vi "Teleop.vi"(10 "Match Info":T1={"Autonomous Elapsed Seconds"=0.0, "TeleOp Elapsed Seconds"=0.0, "Disabled Elapsed Seconds"=0.0, "Visited Autonomous"=FALSE, "Visited TeleOp"=FALSE, "Visited Disabled"=FALSE, "Autonomous Settings"={"Autonomous Style"=enum."Independent", "VI Refnum"=refnum}}, 11 "Call Context":T2) -> ()   [LabVIEW 2013]
doc: "This VI is called for each TeleOp packet received from the DS where the robot is not disabled. It is often used to read from the joysticks and update I/O or to update setpoints for timed control loops. It should complete and return within 20 milliseconds or it may miss DS packets."
uses:
  <vilib>/Rock Robotics/WPI/DriverStation/WPI_DriverStationDerivedRobotMode.ctl
  <vilib>/Rock Robotics/WPI/DriverStation/WPI_DriverStationMatch Info.ctl
  Robot Global Data.vi
  <vilib>/Rock Robotics/WPI/Joystick/WPI_JoystickGetSetRefNum.vi
  <vilib>/Rock Robotics/WPI/RobotDrive/WPI_RobotDriveGetSetRefNum.vi
panel:
  in  "last switch 2":bool
  in  "toggle on/off internal 2":bool=TRUE
  out "toggle on/off 2":bool=TRUE
  out "axis 1 (x) 2":dbl
  out "axis 2 (y) 2":dbl
  out "toggle on/off":bool=TRUE
  in  "toggle on/off internal":bool=TRUE
  in  "last switch":bool
  out "axis 1 (x)":dbl
  out "axis 2 (y)":dbl
  out "Numeric 1":dbl(slide) scale=0.0..100.0
  out "Boolean 2":bool
  out "Boolean 1":bool
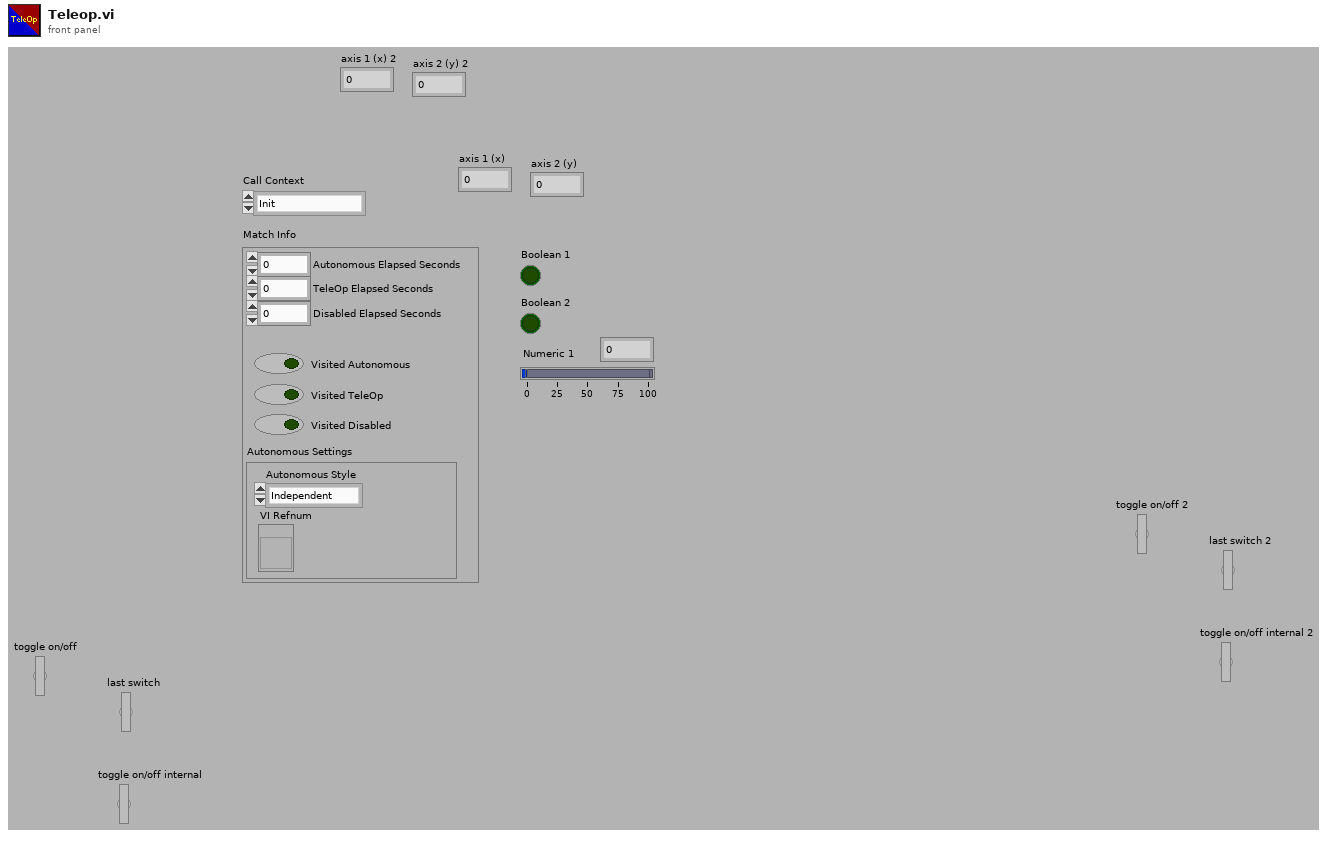
[diagram p1: front panel]
types:
  T1 = typedef "WPI_DriverStationMatch Info.ctl" = cluster{"Autonomous Elapsed Seconds":dbl, "TeleOp Elapsed Seconds":dbl, "Disabled Elapsed Seconds":dbl, "Visited Autonomous":bool, "Visited TeleOp":bool, "Visited Disabled":bool, "Autonomous Settings":cluster{"Autonomous Style":enum16{"Iterative", "Independent"}, "VI Refnum":refnum<vi>}}
  T2 = typedef "WPI_DriverStationDerivedRobotMode.ctl" = enum16{"Init", "Execute", "Stop"}
  T3 = typedef "WPI_JoystickDevRef.ctl" = cluster{"Device":T4}
  T4 = typedef "WPI_JoystickDeviceEnum.ctl" = enum16{"USB 1", "USB 2", "USB 3", "USB 4", "Kinect 1", "Kinect 2"}
  T5 = typedef "WPI_JoystickButtonState.ctl" = cluster{"Button 1":bool, "Button 2":bool, "Button 3":bool, "Button 4":bool, "Button 5":bool, "Button 6":bool, "Button 7":bool, "Button 8":bool, "Button 9":bool, "Button 10":bool, "Button 11":bool, "Button 12":bool}
  T6 = typedef "WPI_RobotDriveDevRef.ctl" = cluster{"DevStatus":errorcluster, "Motors[]":T7[], "Square Inputs":bool, "Max Output":dbl, "Isochronous":bool}
  T7 = typedef "WPI_MotorControlDeviceRef.ctl" = cluster{"DeviceStatus":errorcluster, "Type":enum16{"PWM", "CAN"}, "PWM":cluster{"Digital Module":T8, "PWM Channel":T9, "DeadBand":T10}, "CAN":cluster{"Device Number":u8, "Control Mode":T11, "Semaphore":T12, "Max Vout":dbl}, "Invert":bool, "TransformRef":T13, "InvTransformRef":T13}
  T8 = typedef "FPGA_TypedefDigitalModule.ctl" = enum16{"Digital Module 1", "Digital Module 2"}
  T9 = typedef "FPGA_DIOPWMChannel.ctl" = enum8{"PWM 1", "PWM 2", "PWM 3", "PWM 4", "PWM 5", "PWM 6", "PWM 7", "PWM 8", "PWM 9", "PWM 10", "Invalid"}
  T10 = typedef "WPI_PWMDeadband.ctl" = cluster{"Name":string, "maxPositivePwm":i32, "minPositivePwm":i32, "centerPwm":i32, "maxNegativePwm":i32, "minNegativePwm":i32, "angularRange":u16}
  T11 = typedef "WPI_CANJaguar_ControlMode.ctl" = enum8{"Percent VBus", "Current", "Speed", "Position", "Voltage"}
  T12 = typedef "Semaphore RefNum" = refnum<k1>
  T13 = typedef "WPI_PWMTransform_ConPane.ctl" = refnum<vi>
  T14 = cluster{"axis 1 (x)":dbl, "axis 2 (y)":dbl, "axis 3 (throttle)":dbl, "axis 4":dbl, "axis 5":dbl, "axis 6":dbl}
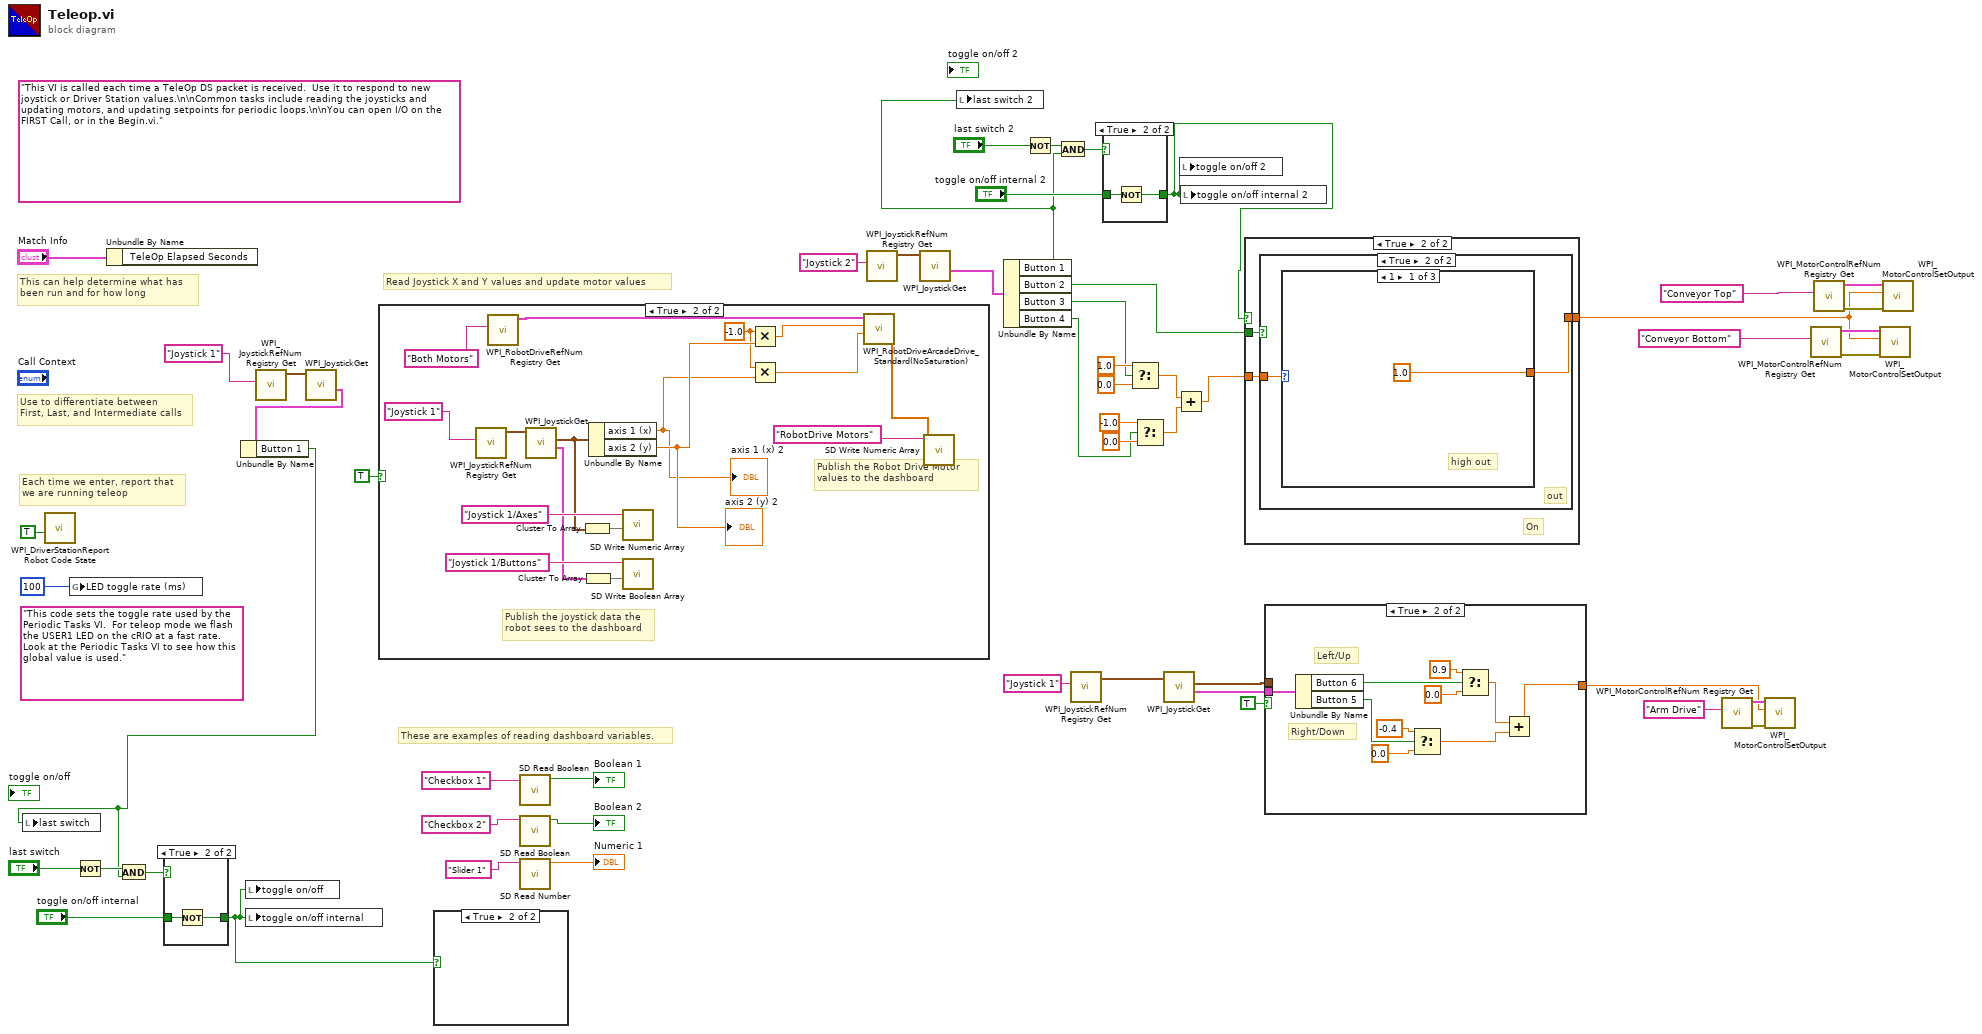
[diagram p0: block diagram]
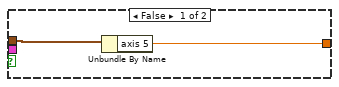
[diagram p3: hidden frame]
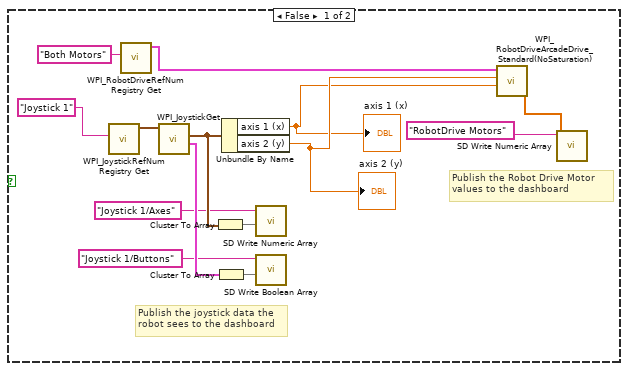
[diagram p6: hidden frame]
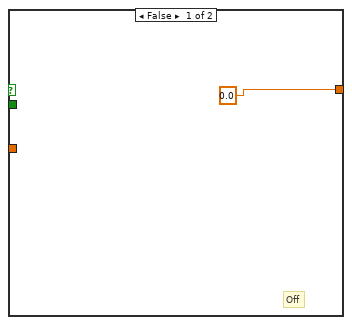
[diagram p7: hidden frame]
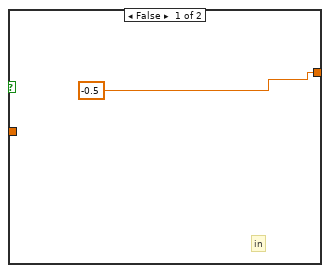
[diagram p8: hidden frame]
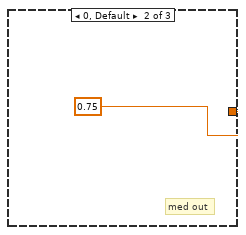
[diagram p9: hidden frame]
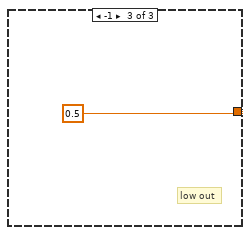
[diagram p10: hidden frame]
diagram:
  (unwired) "This code sets the toggle rate used by the Periodic Tasks VI.  For teleop mode we flash the USER1 LED on the cRIO at a fast rate.  Look at the Periodic Tasks VI to see how this global value is used."
  (unwired) "This VI is called each time a TeleOp DS packet is received.  Use it to respond to new joystick or Driver Station values.\n\nCommon tasks include reading the joysticks and updating motors, and updating setpoints for periodic loops.\n\nYou can open I/O on the FIRST Call, or in the Begin.vi."
  # "These are examples of reading dashboard variables."
  # "Each time we enter, report that\nwe are running teleop"
  # "Use to differentiate between\nFirst, Last, and Intermediate calls"
  # "This can help determine what has\nbeen run and for how long"
  # "Read Joystick X and Y values and update motor values"
  n1 = call <vilib>:"WPI_DriverStationReport Robot Code State.vi"("TeleOp"=TRUE ("Autonomous")) -> ()  [unwired: 10 in, 1 out]
  n2 = global write "Robot Global Data.vi" "LED toggle rate (ms)"(u32 100 ("LED ms toggle rate")) -> ()
  n3 = Not(x="last switch") -> (.not. x?=w25:bool)
  n4 = Unbundle By Name("Match Info") -> ()  [unwired: 1 out]
  n5 = call <vilib>:"WPI_JoystickRefNum Registry Get.vi"("refnum name"="Joystick 1") -> ("JoystickDevRef"=w29:T3)  [unwired: 1 in, 9 out]
  n6 = call <vilib>:"WPI_JoystickGet.vi"("JoystickDevRef"=w29) -> ("Buttons"=w27:T5)  [unwired: 1 in, 5 out]
  n7 = Unbundle By Name(w27) -> ("Button 1"=w22:bool)
  n8 = local write "last switch"(w22) -> ()
  n9 = And(x=w25, y=w22) -> (x .and. y?=w24:bool)
  n10 = case shown="True" w24 {
    tunnel: "toggle on/off internal" -> [w55 w57]
    tunnel: [w55 w56] -> w13
    frame False {
    }
    frame True {
      n11 = Not(x=w57) -> (.not. x?=w56:bool)
    }
  }
  n12 = local write "toggle on/off"(w13) -> ()
  n13 = local write "toggle on/off internal"(w13) -> ()
  n14 = case shown="True" TRUE {
    frame False {
      # "Publish the Robot Drive Motor\nvalues to the dashboard"
      # "Publish the joystick data the\nrobot sees to the dashboard"
      n15 = call <vilib>:"WPI_JoystickRefNum Registry Get.vi"("refnum name"="Joystick 1") -> ("JoystickDevRef"=w70:T3)  [unwired: 1 in, 9 out]
      n16 = call <vilib>:"WPI_RobotDriveRefNum Registry Get.vi"("refnum name"="Both Motors") -> ("RobotDriveDevRef"=w60:T6)  [unwired: 9 in, 1 out]
      n17 = call <vilib>:"WPI_JoystickGet.vi"("JoystickDevRef"=w70) -> ("Buttons"=w69:T5, "Axes"=w66:T14)  [unwired: 1 in, 4 out]
      n18 = Cluster To Array(cluster=w66) -> (array=w65:dbl[])
      n19 = Cluster To Array(cluster=w69) -> (array=w68:bool[])
      n20 = Unbundle By Name(w66) -> ("axis 1 (x)"=w58:dbl, "axis 2 (y)"=w59:dbl)
      "axis 2 (y)" <- w59
      "axis 1 (x)" <- w58
      n21 = call <vilib>:"SD Write Numeric Array.vi"("Numeric Array"=w65, "Name"="Joystick 1/Axes") -> ()  [unwired: 8 in, 2 out]
      n22 = call <vilib>:"SD Write Boolean Array.vi"("Boolean Array"=w68, "Name"="Joystick 1/Buttons") -> ()  [unwired: 8 in, 2 out]
      n23 = call <vilib>:"WPI_RobotDriveArcadeDrive_Standard(NoSaturation).vi"("Y axis value"=w58, "X axis value"=w59, "RobotDriveDevRef"=w60) -> ("Motor Values"=w62:dbl[])  [unwired: 1 in, 7 out]
      n24 = call <vilib>:"SD Write Numeric Array.vi"("Numeric Array"=w62, "Name"="RobotDrive Motors") -> ()  [unwired: 8 in, 2 out]
    }
    frame True {
      w73 = -1.0 ("x")
      # "Publish the Robot Drive Motor\nvalues to the dashboard"
      # "Publish the joystick data the\nrobot sees to the dashboard"
      n25 = call <vilib>:"WPI_JoystickRefNum Registry Get.vi"("refnum name"="Joystick 1") -> ("JoystickDevRef"=w78:T3)  [unwired: 1 in, 9 out]
      n26 = call <vilib>:"WPI_RobotDriveRefNum Registry Get.vi"("refnum name"="Both Motors") -> ("RobotDriveDevRef"=w88:T6)  [unwired: 9 in, 1 out]
      n27 = call <vilib>:"WPI_JoystickGet.vi"("JoystickDevRef"=w78) -> ("Buttons"=w79:T5, "Axes"=w82:T14)  [unwired: 1 in, 4 out]
      n28 = Cluster To Array(cluster=w82) -> (array=w83:dbl[])
      n29 = Cluster To Array(cluster=w79) -> (array=w80:bool[])
      n30 = Unbundle By Name(w82) -> ("axis 1 (x)"=w72:dbl, "axis 2 (y)"=w76:dbl)
      "axis 2 (y) 2" <- w76
      "axis 1 (x) 2" <- w72
      n31 = call <vilib>:"SD Write Numeric Array.vi"("Numeric Array"=w83, "Name"="Joystick 1/Axes") -> ()  [unwired: 8 in, 2 out]
      n32 = call <vilib>:"SD Write Boolean Array.vi"("Boolean Array"=w80, "Name"="Joystick 1/Buttons") -> ()  [unwired: 8 in, 2 out]
      n33 = Multiply(x=w73, y=w76) -> (x*y=w75:dbl)
      n34 = Multiply(x=w73, y=w72) -> (x*y=w74:dbl)
      n35 = call <vilib>:"WPI_RobotDriveArcadeDrive_Standard(NoSaturation).vi"("Y axis value"=w74, "X axis value"=w75, "RobotDriveDevRef"=w88) -> ("Motor Values"=w86:dbl[])  [unwired: 1 in, 7 out]
      n36 = call <vilib>:"SD Write Numeric Array.vi"("Numeric Array"=w86, "Name"="RobotDrive Motors") -> ()  [unwired: 8 in, 2 out]
    }
  }
  n37 = case shown="True" w13 {
    frame False {
    }
    frame True {
    }
  }
  n38 = call <vilib>:"SD Read Boolean.vi"("Name"="Checkbox 1" ("refnum name")) -> ("Boolean"=→"Boolean 1":bool)  [unwired: 8 in, 2 out]
  n39 = call <vilib>:"SD Read Boolean.vi"("Name"="Checkbox 2" ("refnum name")) -> ("Boolean"=→"Boolean 2":bool)  [unwired: 8 in, 2 out]
  n40 = call <vilib>:"SD Read Number.vi"("Name"="Slider 1" ("refnum name")) -> ("Numeric"=→"Numeric 1":dbl)  [unwired: 8 in, 2 out]
  n41 = call <vilib>:"WPI_JoystickRefNum Registry Get.vi"("refnum name"="Joystick 2") -> ("JoystickDevRef"=w39:T3)  [unwired: 9 in, 1 out]
  n42 = call <vilib>:"WPI_JoystickGet.vi"("JoystickDevRef"=w39) -> ("Buttons"=w37:T5)  [unwired: 4 in, 2 out]
  n43 = Unbundle By Name(w37) -> ("Button 1"=w4:bool, "Button 2"=w14:bool, "Button 3"=w1:bool, "Button 4"=w2:bool)
  n44 = local write "last switch 2"(w4) -> ()
  n45 = Not(x="last switch 2") -> (.not. x?=w6:bool)
  n46 = And(x=w6, y=w4) -> (x .and. y?=w7:bool)
  n47 = call <vilib>:"WPI_JoystickRefNum Registry Get.vi"("refnum name"="Joystick 1") -> ("JoystickDevRef"=w44:T3)  [unwired: 9 in, 1 out]
  n48 = case shown="True" w7 {
    tunnel: "toggle on/off internal 2" -> [w89 w91]
    tunnel: [w89 w90] -> w3
    frame False {
    }
    frame True {
      n49 = Not(x=w91) -> (.not. x?=w90:bool)
    }
  }
  n50 = Select(t=1.0, s=w1, f=0.0) -> (s? t:f=w16:dbl)
  n51 = Select(t=-1.0, s=w2, f=0.0) -> (s? t:f=w17:dbl)
  n52 = call <vilib>:"WPI_JoystickGet.vi"("JoystickDevRef"=w44) -> ("Buttons"=w43:T5, "Axes"=w10:T14)  [unwired: 4 in, 1 out]
  n53 = Add(x=w16, y=w17) -> (x+y=w15:dbl)
  n54 = local write "toggle on/off 2"(w3) -> ()
  n55 = local write "toggle on/off internal 2"(w3) -> ()
  n56 = case shown="True" w3 {
    tunnel: [0.0 ("f") w94] -> w30
    tunnel: w15 -> [_ w95]
    tunnel: w14 -> [_ w93]
    frame False {
      # "Off"
    }
    frame True {
      # "On"
      n57 = case shown="True" w93 {
        tunnel: w95 -> [_ w98]
        tunnel: [-0.5 ("t") w97] -> w94
        frame False {
          # "in"
        }
        frame True {
          # "out"
          n58 = case shown="1" w98 {
            tunnel: [1.0 ("t") 0.75 ("t") 0.5 ("f")] -> w97
            frame 1 {
              # "high out"
            }
            frame 0, Default {
              # "med out"
            }
            frame -1 {
              # "low out"
            }
          }
        }
      }
    }
  }
  n59 = case shown="True" TRUE {
    tunnel: w43 -> [_ w113]
    tunnel: w10 -> [w103 _]
    tunnel: [w102 w104] -> w9
    frame False {
      n60 = Unbundle By Name(w103) -> ("axis 5"=w102:dbl)
    }
    frame True {
      # "Right/Down"
      # "Left/Up"
      n61 = Unbundle By Name(w113) -> ("Button 6"=w112:bool, "Button 5"=w111:bool)
      n62 = Select(t=-0.4, s=w111, f=0.0) -> (s? t:f=w106:dbl)
      n63 = Select(t=0.9, s=w112, f=0.0) -> (s? t:f=w105:dbl)
      n64 = Add(x=w105, y=w106) -> (x+y=w104:dbl)
    }
  }
  n65 = call <vilib>:"WPI_MotorControlRefNum Registry Get.vi"("refnum name"="Arm Drive") -> ("error out"=w42:errorcluster, "MotorControlDevRef"=w41:T7)  [unwired: 9 in]
  n66 = call <vilib>:"WPI_MotorControlSetOutput.vi"("error in (no error)"=w42, "Output"=w9, "MotorControlDevRef"=w41) -> ()  [unwired: 6 in, 3 out]
  n67 = call <vilib>:"WPI_MotorControlRefNum Registry Get.vi"("refnum name"="Conveyor Bottom") -> ("error out"=w33:errorcluster, "MotorControlDevRef"=w32:T7)  [unwired: 9 in]
  n68 = call <vilib>:"WPI_MotorControlRefNum Registry Get.vi"("refnum name"="Conveyor Top") -> ("error out"=w34:errorcluster, "MotorControlDevRef"=w35:T7)  [unwired: 9 in]
  n69 = call <vilib>:"WPI_MotorControlSetOutput.vi"("error in (no error)"=w33, "Output"=w30, "MotorControlDevRef"=w32) -> ()  [unwired: 6 in, 3 out]
  n70 = call <vilib>:"WPI_MotorControlSetOutput.vi"("error in (no error)"=w34, "Output"=w30, "MotorControlDevRef"=w35) -> ()  [unwired: 6 in, 3 out]
